vi "Create from SFTP Directory.vi"(8 "Error In":errorcluster, 11 "SFTP Directory":refnum<class "SFTP Directory.lvclass">) -> (0 "Error Out":errorcluster, 3 "SFTP Attributes":refnum<class "SFTP Attributes.lvclass">)   [LabVIEW 2018, in "Toolkit.lvlib" / "SFTP Attributes.lvclass"]
uses:
  SFTP Attributes.lvclass
  SFTP Directory/SFTP Directory.lvclass
  SFTP Directory/SFTP Directory.lvclass/SFTP Directory.ctl
  SFTP/SFTP.lvclass/SFTP.ctl
  SSH/SSH.lvclass
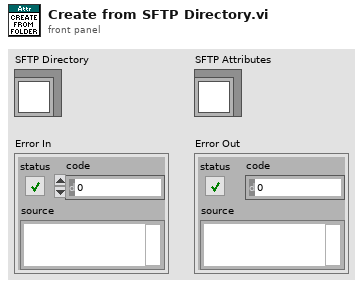
[diagram p1: front panel]
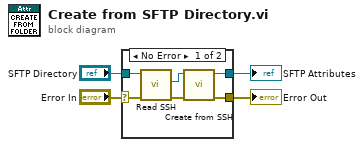
[diagram p0: block diagram]
diagram:
  n1 = case shown="No Error" "Error In" {
    selector: "Error In" -> [w5 w11]
    tunnel: [w9 w11] -> w3
    tunnel: [w10 _] -> w2
    tunnel: "SFTP Directory" -> [w8 _]
    frame No Error {
      n2 = call "Read SSH.vi"("Error In"=w5, "SFTP Directory In"=w8) -> ("Error Out"=w6:errorcluster, "SSH"=w7:refnum<class "SSH.lvclass">)  [unwired: 7 in, 1 out]
      n3 = call "Create from SSH.vi"("Error In"=w6, "SSH"=w7) -> ("Error Out"=w9:errorcluster, "SFTP Attributes"=w10:refnum<class "SFTP Attributes.lvclass">)  [unwired: 8 in]
    }
    frame Error {
    }
  }
  "Error Out" <- w3
  "SFTP Attributes" <- w2
